vi "PassNill.vi"(8 "Error In":errorcluster) -> (0 "Error Out":errorcluster)   [LabVIEW 2013, in "main.lvlib"]
uses:
  main.lvlib
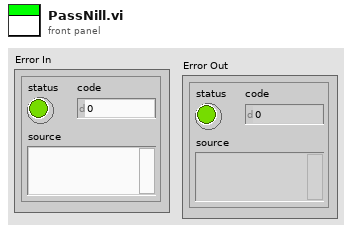
[diagram p1: front panel]
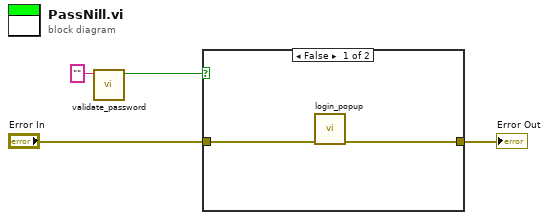
[diagram p0: block diagram]
diagram:
  n1 = call "validate_password.vi"("Password"="") -> ("Accept"=w1:bool)  [unwired: 10 in]
  n2 = case shown="False" w1 {
    tunnel: "Error In" -> [w6 w7]
    tunnel: [w5 w7] -> w3
    frame False {
      n3 = call "login_popup.vi"("Error In"=w6) -> ("Error Out"=w5:errorcluster)  [unwired: 10 in]
    }
    frame True {
    }
  }
  "Error Out" <- w3
